vi "Matrix_SetColumn.vi"(9 "Fill Vector":T1, 10 "Column":i32, 11 "input matrix":T1) -> (0 "Error":bool, 3 "output matrix":T1)   [LabVIEW 2019, in "Trajectory_Library.lvlib"]
doc: "Sets a column to a given column vector.\n \n\nInputs:\n - input matrix -- The input matrix\n - column -- The column to set.\n - val -- The column vector to set the given row to.\n\nOutputs:\n - output matrix -- the resulting matrix\n - error -- If TRUE, an error occured."
uses:
  Trajectory_Library.lvlib
  <vilib>/Analysis/Matrix/Datatypes/RealMatrix.ctl
  MatBuilder_Create.vi
  <vilib>/Analysis/Matrix/NI_Matrix.lvlib
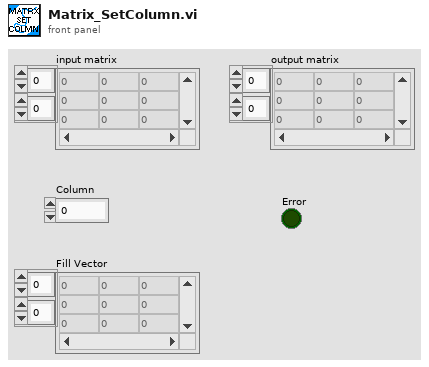
[diagram p1: front panel]
types:
  T1 = typedef "NI_Matrix.lvlib/RealMatrix.ctl" = dbl[][]
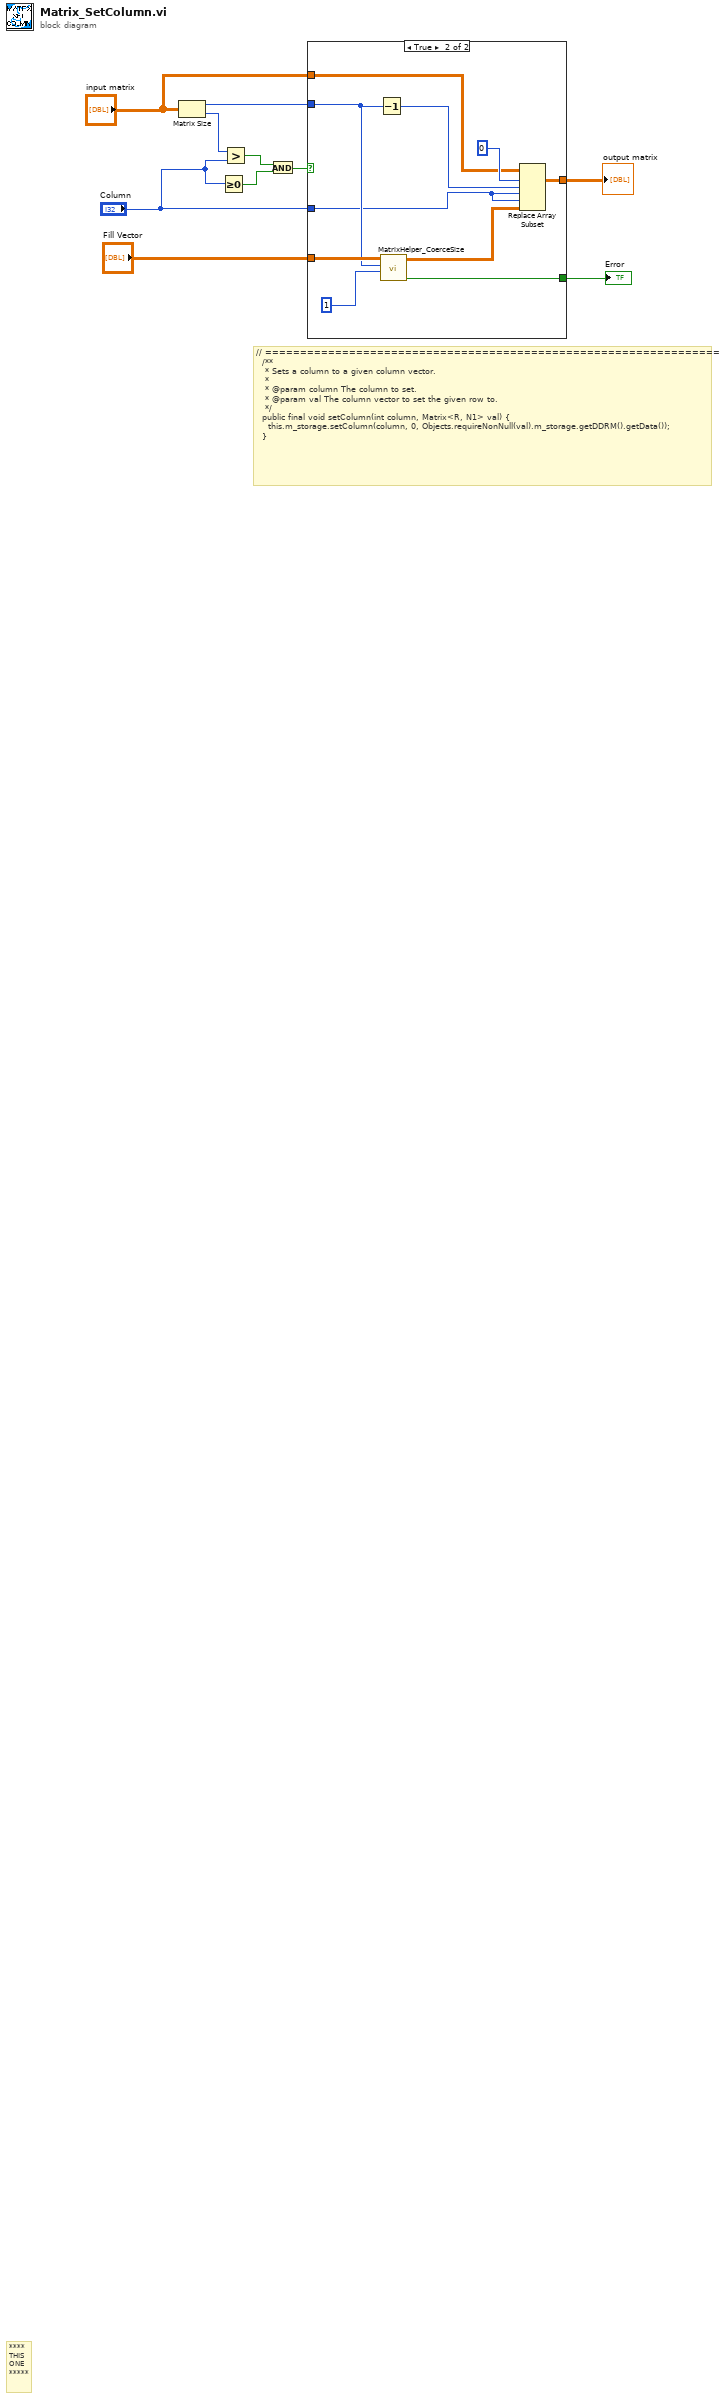
[diagram p0: block diagram]
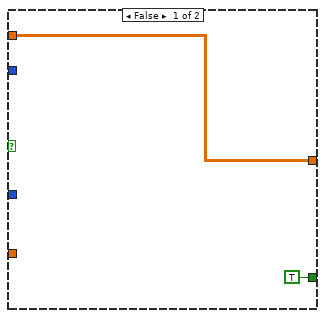
[diagram p2: hidden frame]
diagram:
  # "// ==================================================================\n  /**\n   * Sets a column to a given column vector.\n   *\n   * @param column The column to set.\n   * @param val The column vector to set the given row to.\n   */\n  public final void setColumn(int column, Matrix<R, N1> val) {\n    this.m_storage.setColumn(column, 0, Objects.requireNonNull(val).m_storage.getDDRM().getData());\n  }"
  # "****\nTHIS\nONE\n*****"
  n1 = Matrix Size(0:"input matrix") -> (1:w4:i32, 2:w3:i32)
  n2 = Greater Or Equal To 0?(x="Column") -> (x >= 0?=w6:bool)
  n3 = Greater?(x=w3, y="Column") -> (0:w7:bool)
  n4 = And(x=w7, y=w6) -> (x .and. y?=w1:bool)
  n5 = case shown="True" w1 {
    tunnel: "Fill Vector" -> [_ w22]
    tunnel: [w11 w17] -> w9
    tunnel: [TRUE ("Coerced") w16] -> w8
    tunnel: "input matrix" -> [w11 w15]
    tunnel: w4 -> [_ w14]
    tunnel: "Column" -> [_ w13]
    frame False {
    }
    frame True {
      n6 = Decrement(x=w14) -> (x-1=w19:i32)
      n7 = call "MatrixHelper_CoerceSize.vi"("Columns"=1, "Rows"=w14, "input matrix"=w22) -> ("Coerced"=w16:bool, "output matrix"=w18:T1)  [unwired: 7 in]
      n8 = Replace Array Subset(array=w15, new element=w18, index (dim 0)=0 ("row 1"), index (dim 1)=w19, index (dim 2)=w13, index (dim 3)=w13) -> (w17:T1)
    }
  }
  "output matrix" <- w9
  "Error" <- w8
